vi "Create from Session.vi"(8 "Error In":errorcluster, 11 "Session":refnum<class "Session.lvclass">) -> (0 "Error Out":errorcluster, 3 "Channel":refnum<class "Channel.lvclass">)   [LabVIEW 2018, in "Toolkit.lvlib" / "Channel.lvclass"]
uses:
  Channel.lvclass
  Session/Session.lvclass
  Session/Session.lvclass/Session.ctl
  SSH/SSH.lvclass/SSH.ctl
  Channel.lvclass/Channel.ctl
  Toolkit.lvlib
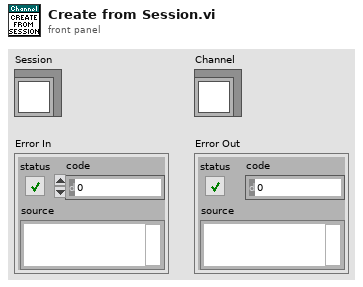
[diagram p1: front panel]
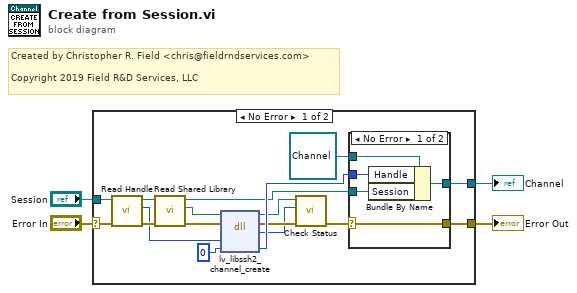
[diagram p0: block diagram]
diagram:
  # "Created by Christopher R. Field <chris@fieldrndservices.com>\n\nCopyright 2019 Field R&D Services, LLC"
  n1 = case shown="No Error" "Error In" {
    selector: "Error In" -> [w19 w29]
    tunnel: [w7 w29] -> w3
    tunnel: "Session" -> [w20 _]
    tunnel: [w21 _] -> w1
    frame No Error {
      n2 = call "Read Handle.vi"("Error In"=w19, "Session In"=w20) -> ("Erorr Out"=w17:errorcluster, "Handle"=w14:u64, "Session Out"=w18:refnum<class "Session.lvclass">)  [unwired: 7 in]
      n3 = call "Read Shared Library.vi"("Error In"=w17, "Session In"=w18) -> ("Erorr Out"=w16:errorcluster, "libssh2lv Shared Library"=w15:path, "Session Out"=w6:refnum<class "Session.lvclass">)  [unwired: 7 in]
      n4 = dll-call lib="libssh2lv.*" fn="lv_libssh2_channel_create"(path in=w15, error in=w16, "session"=w14, "handle"=u64 0) -> (path out=w9:path, error out=w11:errorcluster, "status"=w10:i32, "handle"=w12:u64)  [unwired: 2 in]
      n5 = call "Check Status.vi"("Error In"=w11, "Status"=w10, "lv-libssh2 Shared Library In"=w9) -> ("Error Out"=w8:errorcluster)  [unwired: 7 in, 1 out]
      n6 = case shown="No Error" w8 {
        selector: w8 -> [w25 w28]
        tunnel: [w22 w27] -> w21
        tunnel: w12 -> [w26 _]
        tunnel: [w25 w28] -> w7
        tunnel: w6 -> [w24 _]
        tunnel: refnum<class "Channel.lvclass"> refnum ("Toolkit.lvlib:Channel.lvclass") -> [w23 w27]
        frame No Error {
          n7 = Bundle By Name(cluster=w23, "Handle"=w26, "Session"=w24) -> (w22:refnum<class "Channel.lvclass">)
        }
        frame Error {
        }
      }
    }
    frame Error {
    }
  }
  "Error Out" <- w3
  "Channel" <- w1
